vi "DependencyViewer AllVIs.vi"   [LabVIEW 2020]
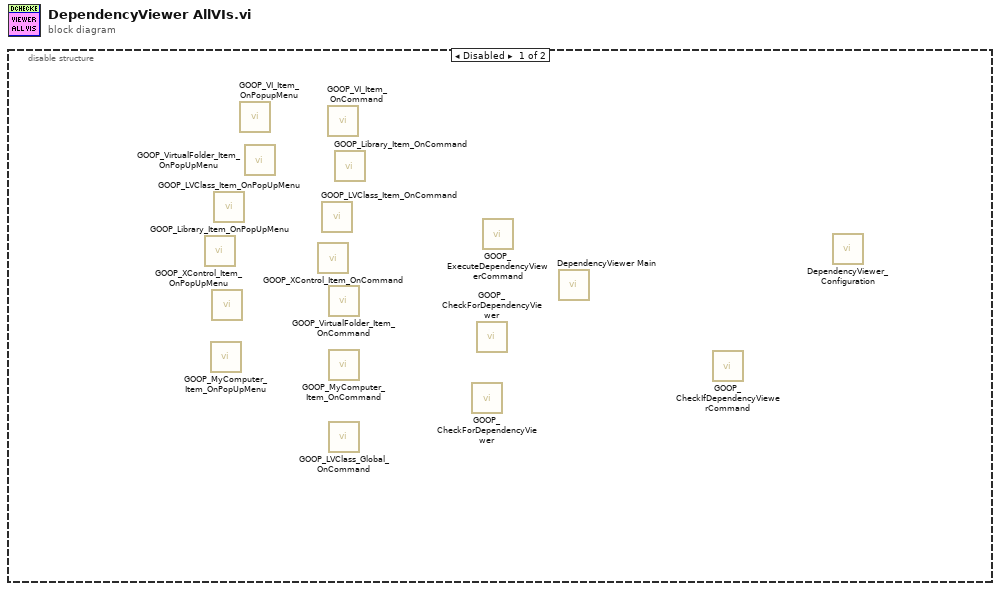
[diagram p0: block diagram]
diagram:
  n1 = disable-structure shown="Disabled" {
    frame Disabled {
      n2 = call <resource>:"GOOP_Library_Item_OnPopUpMenu.vi"() -> ()  [unwired: 12 in]
      n3 = call <resource>:"GOOP_MyComputer_Item_OnPopUpMenu.vi"() -> ()  [unwired: 12 in]
      n4 = call <resource>:"GOOP_XControl_Item_OnPopUpMenu.vi"() -> ()  [unwired: 12 in]
      n5 = call <resource>:"GOOP_LVClass_Item_OnPopUpMenu.vi"() -> ()  [unwired: 12 in]
      n6 = call <resource>:"GOOP_VI_Item_OnPopupMenu.vi"() -> ()  [unwired: 12 in]
      n7 = call <resource>:"GOOP_VirtualFolder_Item_OnPopUpMenu.vi"() -> ()  [unwired: 12 in]
      n8 = call <resource>:"GOOP_XControl_Item_OnCommand.vi"() -> ()  [unwired: 12 in]
      n9 = call <resource>:"GOOP_LVClass_Item_OnCommand.vi"() -> ()  [unwired: 12 in]
      n10 = call <resource>:"GOOP_VI_Item_OnCommand.vi"() -> ()  [unwired: 12 in]
      n11 = call <resource>:"GOOP_VirtualFolder_Item_OnCommand.vi"() -> ()  [unwired: 12 in]
      n12 = call <resource>:"GOOP_MyComputer_Item_OnCommand.vi"() -> ()  [unwired: 12 in]
      n13 = call <resource>:"GOOP_LVClass_Global_OnCommand.vi"() -> ()  [unwired: 12 in]
      n14 = call <resource>:"GOOP_Library_Item_OnCommand.vi"() -> ()  [unwired: 12 in]
      n15 = call <resource>:"GOOP_CheckForDependencyViewer.vi"() -> ()  [unwired: 9 in, 3 out]
      n16 = call <resource>:"GOOP_CheckForDependencyViewer.vi"() -> ()  [unwired: 9 in, 3 out]
      n17 = call <resource>:"GOOP_ExecuteDependencyViewerCommand.vi"() -> ()  [unwired: 12 in]
      n18 = call <resource>:"DependencyViewer Main.vi"() -> ()  [unwired: 12 in]
      n19 = call <resource>:"GOOP_CheckIfDependencyViewerCommand.vi"() -> ()  [unwired: 10 in, 2 out]
      n20 = call <resource>:"DependencyViewer_Configuration.vi"() -> ()  [unwired: 11 in, 1 out]
    }
    frame Enabled {
    }
  }
